vi "VTM_WT1.vi"() -> ()   [LabVIEW 2012]
uses:
  <vilib>/xnet/xnet.llb/XNET Frame CAN.ctl
  <vilib>/xnet/xnet.llb/XNET Frame Type CAN.ctl
  <vilib>/xnet/xnet.llb/XNET Create Session (Frame Input Single-point).vi
  <vilib>/xnet/xnet.llb/XNET Read (Frame CAN).vi
panel:
  in  "Logging":bool
  in  "Tab Control":T1(tab)
  out "MAP":dbl(knob) caption="psi" scale=-15.0..5.0 scale format="%#_2g"
  out "Lambda":dbl(graph)
  out "IAT (F)":dbl(slide) scale=0.0..110.0
  out "ECU Internal":bool
  out "EGT (F)":u16(slide) scale=500.0..2000.0
  out "RPM":dbl(knob) caption="x1000" scale=0.0..11.0 scale format="%#_3g"
  out "ET (F)":dbl(slide) scale=0.0..230.0
  out "Bat (V)":dbl(slide) scale=0.0..15.0
  out "TP (%)":dbl(slide) scale=0.0..100.0
  out "Engine Temp":bool
  out "Battery Voltage":bool
  out "Oil Pressure":u16
  out "Fuel Pressure":u16
  out "Exhaust Gas Temp":bool
  out "RPM>=500?":bool
  out "Table of Weighted Averages":dbl[][](array[numeric])
  out "data":T2[](array[typedef]) {"payload" format="%x"; "timestamp" format="%<%.7X\n%x>T"; "type" items=["CAN Data"=0, "CAN Remote"=1, "Delay"=224]; "identifier" format="%x"}
  out "ECU Internal Temp (F)":dbl(slide) scale=0.0..150.0
  out "Problem?":bool
  out "timestamp":timestamp
  in  "Select Interface":refnum<k21>
  in  "stop":bool
  # "Virginia Tech Motorsports Wireless Telemetry VI"
  # "Shaishav Parekh"
  # "Warning Lights:"
  # "Green = Good, Red = Bad"
  # "FP, OP = dials\nSlip = Avg value for front / Avg value for rear ->\nChart"
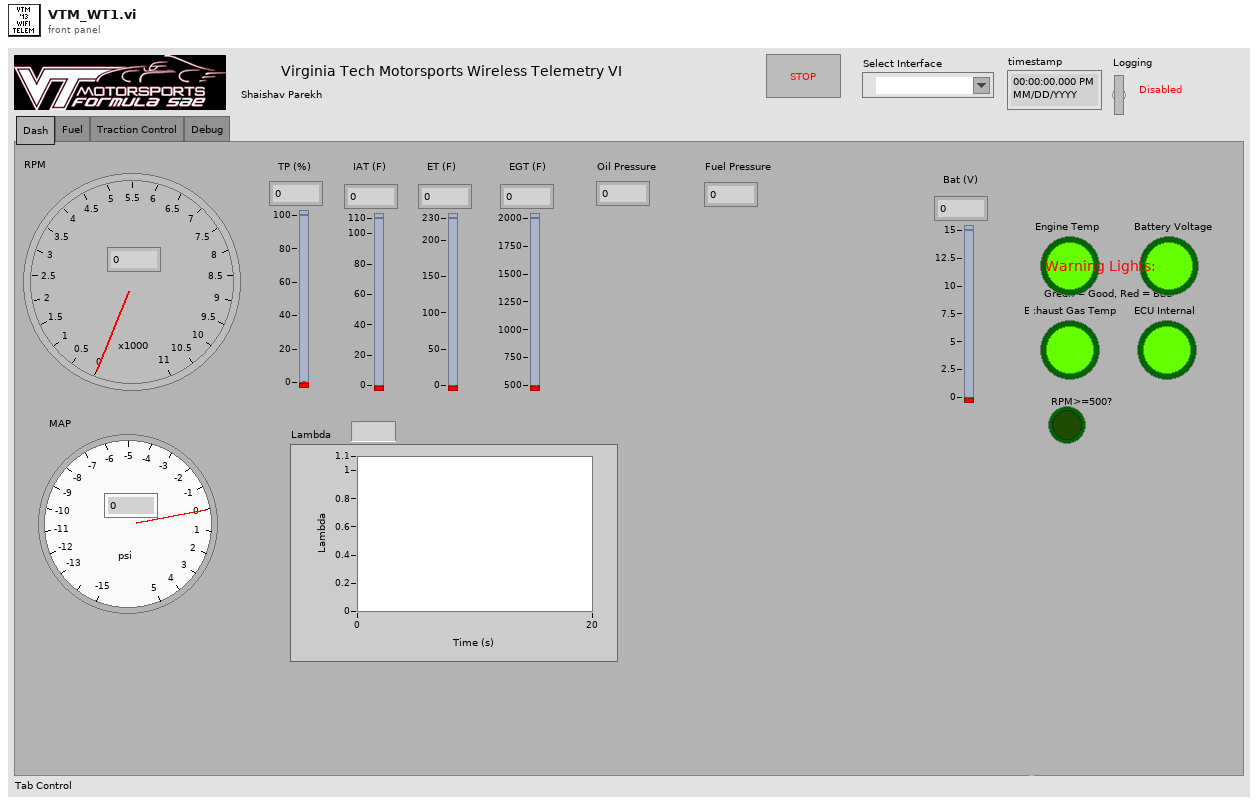
[diagram p1: front panel]
types:
  T1 = enum32{"Dash", "Fuel", "Traction Control", "Debug"}
  T2 = typedef "XNET Frame CAN.ctl" = cluster{"timestamp":timestamp, "payload":u8[], "identifier":u32, "type":T3, "extended?":bool, "echo?":bool}
  T3 = typedef "XNET Frame Type CAN.ctl" = u8
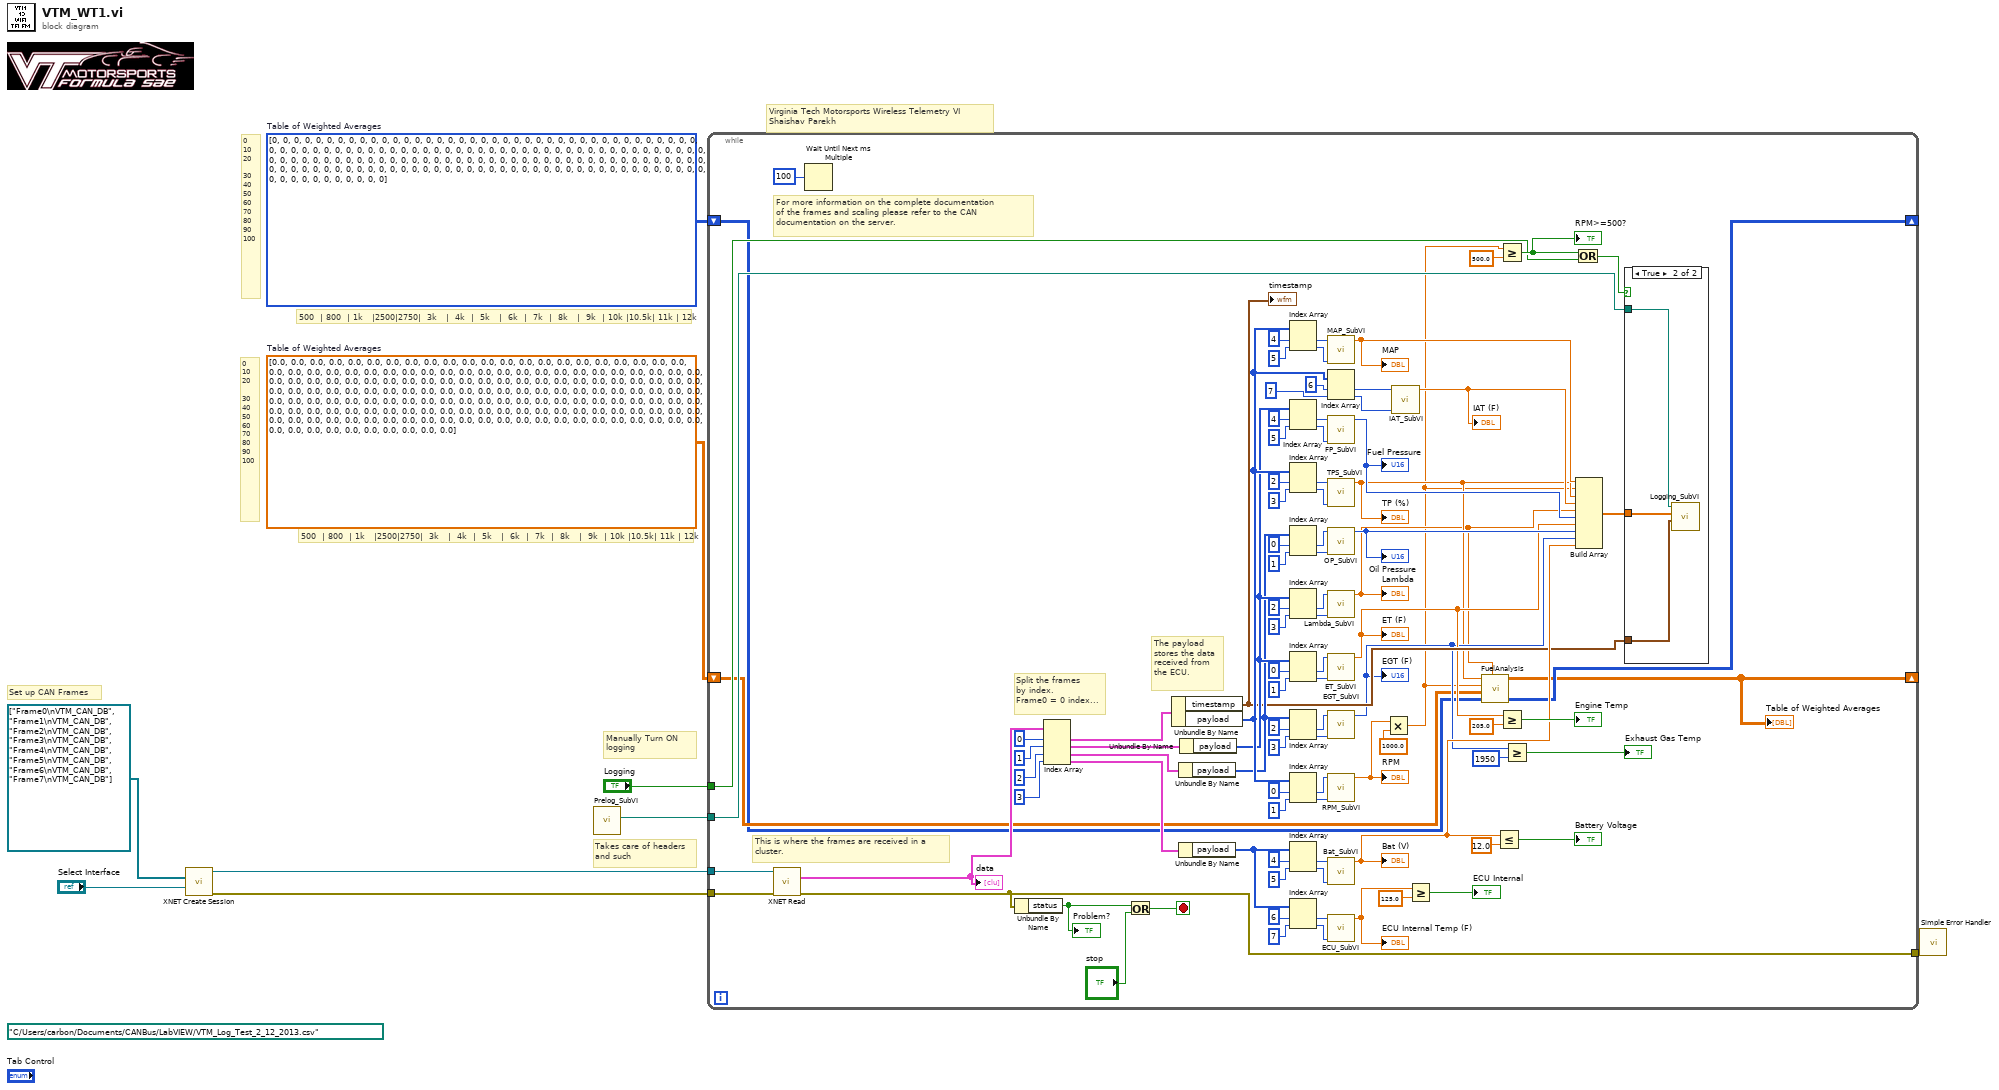
[diagram p0: block diagram]
diagram:
  w1 = i32[][] [[0, 0, 0, 0, 0, 0, 0, 0, 0, 0, 0, 0, 0, 0, 0, 0, 0], [0, 0, 0, 0, 0, 0, 0, 0, 0, 0, 0, 0, 0, 0, 0, 0, 0], [0, 0, 0, 0, 0, 0, 0, 0, 0, 0, 0, 0, 0, 0, 0, 0, 0], [0, 0, 0, 0, 0, 0, 0, 0, 0, 0, 0, 0, 0, 0, 0, 0, 0], [0, 0, 0, 0, 0, 0, 0, 0, 0, 0, 0, 0, 0, 0, 0, 0, 0], [0, 0, 0, 0, 0, 0, 0, 0, 0, 0, 0, 0, 0, 0, 0, 0, 0], [0, 0, 0, 0, 0, 0, 0, 0, 0, 0, 0, 0, 0, 0, 0, 0, 0], [0, 0, 0, 0, 0, 0, 0, 0, 0, 0, 0, 0, 0, 0, 0, 0, 0], [0, 0, 0, 0, 0, 0, 0, 0, 0, 0, 0, 0, 0, 0, 0, 0, 0], [0, 0, 0, 0, 0, 0, 0, 0, 0, 0, 0, 0, 0, 0, 0, 0, 0]]  # Table of Weighted Averages
  w2 = dbl[][] [[0.0, 0.0, 0.0, 0.0, 0.0, 0.0, 0.0, 0.0, 0.0, 0.0, 0.0, 0.0, 0.0, 0.0, 0.0, 0.0, 0.0], [0.0, 0.0, 0.0, 0.0, 0.0, 0.0, 0.0, 0.0, 0.0, 0.0, 0.0, 0.0, 0.0, 0.0, 0.0, 0.0, 0.0], [0.0, 0.0, 0.0, 0.0, 0.0, 0.0, 0.0, 0.0, 0.0, 0.0, 0.0, 0.0, 0.0, 0.0, 0.0, 0.0, 0.0], [0.0, 0.0, 0.0, 0.0, 0.0, 0.0, 0.0, 0.0, 0.0, 0.0, 0.0, 0.0, 0.0, 0.0, 0.0, 0.0, 0.0], [0.0, 0.0, 0.0, 0.0, 0.0, 0.0, 0.0, 0.0, 0.0, 0.0, 0.0, 0.0, 0.0, 0.0, 0.0, 0.0, 0.0], [0.0, 0.0, 0.0, 0.0, 0.0, 0.0, 0.0, 0.0, 0.0, 0.0, 0.0, 0.0, 0.0, 0.0, 0.0, 0.0, 0.0], [0.0, 0.0, 0.0, 0.0, 0.0, 0.0, 0.0, 0.0, 0.0, 0.0, 0.0, 0.0, 0.0, 0.0, 0.0, 0.0, 0.0], [0.0, 0.0, 0.0, 0.0, 0.0, 0.0, 0.0, 0.0, 0.0, 0.0, 0.0, 0.0, 0.0, 0.0, 0.0, 0.0, 0.0], [0.0, 0.0, 0.0, 0.0, 0.0, 0.0, 0.0, 0.0, 0.0, 0.0, 0.0, 0.0, 0.0, 0.0, 0.0, 0.0, 0.0], [0.0, 0.0, 0.0, 0.0, 0.0, 0.0, 0.0, 0.0, 0.0, 0.0, 0.0, 0.0, 0.0, 0.0, 0.0, 0.0, 0.0]]  # Table of Weighted Averages
  (unwired) path "C:/Users/carbon/Documents/CANBus/LabVIEW/VTM_Log_Test_2_12_2013.csv" ("file path (dialog if empty)")
  # "0\n10\n20\n\n30\n40\n50\n60\n70\n80\n90\n100"
  # "500  | 800  | 1k   |2500|2750|  3k   |  4k  |  5k   |  6k  |  7k  |  8k   |  9k  | 10k |10.5k| 11k | 12k"
  # "0\n10\n20\n\n30\n40\n50\n60\n70\n80\n90\n100"
  # "500  | 800  | 1k   |2500|2750|  3k   |  4k  |  5k   |  6k  |  7k  |  8k   |  9k  | 10k |10.5k| 11k | 12k"
  # "Manually Turn ON \nlogging"
  # "Set up CAN Frames"
  # "Takes care of headers\nand such"
  # "Virginia Tech Motorsports Wireless Telemetry VI\nShaishav Parekh"
  n1 = call-poly <vilib>:"XNET Create Session.vi"("frame list"=refnum<k21>[] ["Frame0\nVTM_CAN_DB", "Frame1\nVTM_CAN_DB", "Frame2\nVTM_CAN_DB", "Frame3\nVTM_CAN_DB", "Frame4\nVTM_CAN_DB", "Frame5\nVTM_CAN_DB", "Frame6\nVTM_CAN_DB", "Frame7\nVTM_CAN_DB"], "interface"="Select Interface") -> ("session out"=w7:refnum<k21>, "error out"=w8:errorcluster)  [unwired: 12 in]
  n2 = call "Prelog_SubVI.vi"() -> ("path"=w3:path)  [unwired: 10 in]
  n3 = while {
    tunnel: w8 -> [w100]
    tunnel: w7 -> [w101]
    tunnel: [w96] -> w6
    tunnel: "Logging" -> [w23]
    tunnel: w3 -> [w25]
    shift-right: [w14] -> _
    shift-left: w1 -> [w15]
    shift-right: [w13] -> _
    shift-left: w2 -> [w16]
    stop <- w99 stop-if-true
    # "The payload\nstores the data\nreceived from\nthe ECU."
    # "For more information on the complete documentation\nof the frames and scaling please refer to the CAN\ndocumentation on the server."
    # "Split the frames\nby index. \nFrame0 = 0 index..."
    # "This is where the frames are received in a \ncluster."
    n4 = call-poly <vilib>:"XNET Read.vi"("session in"=w101, "error in (no error)"=w100) -> ("data"=w94:T2[], "error out"=w96:errorcluster)  [unwired: 10 in, 2 out]
    "data" <- w94
    n5 = Wait Until Next ms Multiple(millisecond multiple=u32 100) -> ()  [unwired: 1 out]
    n6 = Unbundle By Name(w96) -> ("status"=w98:bool)
    "Problem?" <- w98
    n7 = Index Array(array=w94, index #1=0 ("index"), index #2=1 ("index"), index #3=2 ("index"), index #4=3 ("index")) -> (element #1=w93:T2, element #2=w88:T2, element #3=w72:T2, element #4=w75:T2)
    n8 = Or(x=w98, y="stop") -> (x .or. y?=w99:bool)
    n9 = Unbundle By Name(w93) -> ("timestamp"=w30:timestamp, "payload"=w57:u8[])
    "timestamp" <- w30
    n10 = Unbundle By Name(w72) -> ("payload"=w42:u8[])
    n11 = Unbundle By Name(w75) -> ("payload"=w66:u8[])
    n12 = Unbundle By Name(w88) -> ("payload"=w48:u8[])
    n13 = Index Array(array=w57, index #1=4 ("index"), index #2=5 ("index")) -> (element #1=w21:u8, element #2=w20:u8)
    n14 = Index Array(array=w48, index #1=4 ("index"), index #2=5 ("index")) -> (element #1=w44:u8, element #2=w45:u8)
    n15 = Index Array(array=w57, index #1=2 ("index"), index #2=3 ("index")) -> (element #1=w85:u8, element #2=w84:u8)
    n16 = Index Array(array=w42, index #1=0 ("index"), index #2=1 ("index")) -> (element #1=w69:u8, element #2=w70:u8)
    n17 = Index Array(array=w48, index #1=2 ("index"), index #2=3 ("index")) -> (element #1=w49:u8, element #2=w50:u8)
    n18 = Index Array(array=w48, index #1=0 ("index"), index #2=1 ("index")) -> (element #1=w80:u8, element #2=w81:u8)
    n19 = Index Array(array=w42, index #1=2 ("index"), index #2=3 ("index")) -> (element #1=w38:u8, element #2=w39:u8)
    n20 = Index Array(array=w57, index #1=0 ("index"), index #2=1 ("index")) -> (element #1=w89:u8, element #2=w22:u8)
    n21 = Index Array(array=w66, index #1=4 ("index"), index #2=5 ("index")) -> (element #1=w76:u8, element #2=w77:u8)
    n22 = Index Array(array=w66, index #1=6 ("index"), index #2=7 ("index")) -> (element #1=w62:u8, element #2=w63:u8)
    n23 = call "MAP_SubVI.vi"("High Byte"=w21, "Low Byte"=w20) -> ("MAP"=w37:dbl)  [unwired: 8 in]
    "MAP" <- w37
    n24 = Index Array(array=w57, index #1=6 ("index"), index #2=7 ("index")) -> (element #1=w53:u8, element #2=w54:u8)
    n25 = call "FP_SubVI.vi"("High Byte"=w44, "Low Byte"=w45) -> ("Fuel Pressure"=w29:u16)  [unwired: 8 in]
    "Fuel Pressure" <- w29
    n26 = call "TPS_SubVI.vi"("High Byte"=w85, "Low Byte"=w84) -> ("TPS"=w18:dbl)  [unwired: 8 in]
    "TP (%)" <- w18
    n27 = call "OP_SubVI.vi"("High Byte"=w69, "Low Byte"=w70) -> ("Oil Pressure"=w33:u16)  [unwired: 8 in]
    "Oil Pressure" <- w33
    n28 = call "Lambda_SubVI.vi"("High Byte"=w49, "Low Byte"=w50) -> ("Lambda"=w17:dbl)  [unwired: 8 in]
    "Lambda" <- w17
    n29 = call "ET_SubVI.vi"("High Byte"=w80, "Low Byte"=w81) -> ("Engine Temp"=w28:dbl)  [unwired: 8 in]
    "ET (F)" <- w28
    n30 = call "EGT_SubVI.vi"("High Byte"=w38, "Low Byte"=w39) -> ("EGT"=w19:u16)  [unwired: 8 in]
    "EGT (F)" <- w19
    n31 = call "RPM_SubVI.vi"("High Byte"=w89, "Low Byte"=w22) -> ("RPM"=w11:dbl)  [unwired: 8 in]
    "RPM" <- w11
    n32 = call "Bat_SubVI.vi"("High Byte"=w76, "Low Byte"=w77) -> ("Battery Voltage"=w32:dbl)  [unwired: 8 in]
    "Bat (V)" <- w32
    n33 = call "ECU_SubVI.vi"("High Byte"=w62, "Low Byte"=w63) -> ("ECU"=w61:dbl)  [unwired: 8 in]
    "ECU Internal Temp (F)" <- w61
    n34 = Multiply(x=w11, y=1000.0) -> (x*y=w12:dbl)
    n35 = call "IAT_SubVI.vi"("High Byte"=w53, "Low Byte"=w54) -> ("IAT"=w34:dbl)  [unwired: 8 in]
    "IAT (F)" <- w34
    n36 = Greater Or Equal?(x=w61, y=125.0) -> (x >= y?=→"ECU Internal":bool)
    n37 = call "FuelAnalysis.vi"("Lambda In"=w17, "Counts - In"=w15, "Table of Weighted Average Values - In"=w16, "RPM"=w12, "Throttle Pos"=w18) -> ("Counts"=w14:i32[][], "Table of Weighted Average Values"=w13:dbl[][])  [unwired: 5 in]
    "Table of Weighted Averages" <- w13
    n38 = Less Or Equal?(x=w32, y=12.0) -> (x <= y?=→"Battery Voltage":bool)
    n39 = Greater Or Equal?(x=w12, y=500.0) -> (x >= y?=w24:bool)
    "RPM>=500?" <- w24
    n40 = Greater Or Equal?(x=w28, y=205.0) -> (x >= y?=→"Engine Temp":bool)
    n41 = Greater Or Equal?(x=w19, y=u16 1950) -> (x >= y?=→"Exhaust Gas Temp":bool)
    n42 = Or(x=w24, y=w23) -> (x .or. y?=w27:bool)
    n43 = Build Array(w37, w12, w18, w34, w17, w29, w28, w33, w19, w32) -> (w31:dbl[])
    n44 = case shown="True" w27 {
      tunnel: w31 -> [_ w108]
      tunnel: w30 -> [_ w107]
      tunnel: w25 -> [_ w106]
      frame False {
      }
      frame True {
        n45 = call "Logging_SubVI.vi"("timestamp"=w107, "Array"=w108, "file path (dialog if empty)"=w106) -> ()  [unwired: 9 in]
      }
    }
  }
  n46 = call <vilib>:"Simple Error Handler.vi"("error in (no error)"=w6) -> ()  [unwired: 4 in, 5 out]
